vi "USRP Config.vi"(0 "USRP Configuration":T6={"USRP RIO Resources"=["USRP-2954"], "reference frequency source"="Internal"}, 5 "rx config":T4={"rf enable 0"=FALSE, "rf config 0"={"antenna"="RX2", "frequency"=2000000000.0, "lo frequency"=-1.0, "level"=0.0}, "rf enable 1"=FALSE, "rf config 1"={"antenna"="RX2", "frequency"=2000000000.0, "lo frequency"=-1.0, "level"=0.0}, "transfer mode"=enum."Finite", "sample rate"=10000000.0, "start trigger"=enum."Immediate"} {"sample rate" format="%#.3pS/s"; "rf config 1"."level" format="%#_gdBm"; "rf config 1"."lo frequency" format="%#.3pHz"; "rf config 1"."frequency" format="%#.3pHz"; "rf config 0"."level" format="%#_gdBm"; "rf config 0"."lo frequency" format="%#.3pHz"; "rf config 0"."frequency" format="%#.3pHz"}, 7 "tx config":T3={"rf enable 0"=FALSE, "rf config 0"={"antenna"="TX1", "frequency"=2000000000.0, "lo frequency"=-1.0, "level"=0.0}, "rf enable 1"=FALSE, "rf config 1"={"antenna"="TX1", "frequency"=2000000000.0, "lo frequency"=-1.0, "level"=0.0}, "transfer mode"=enum."Finite", "sample rate"=10000000.0, "start trigger"=enum."Immediate"} {"sample rate" format="%#.3pS/s"; "rf config 0"."level" format="%#_gdBm"; "rf config 0"."lo frequency" format="%#.3pHz"; "rf config 0"."frequency" format="%#.3pHz"; "rf config 1"."level" format="%#_gdBm"; "rf config 1"."lo frequency" format="%#.3pHz"; "rf config 1"."frequency" format="%#.3pHz"}, 11 "error in (no error)":errorcluster, 12 "Rx?":bool) -> (2 "tx channels":T1={"tx config"={"channel configuration"=[{"channel enable"=FALSE, "channel configuration"={"antenna"="TX1", "frequency"=2000000000.0, "lo frequency"=-1.0, "level"=0.0}}, {"channel enable"=FALSE, "channel configuration"={"antenna"="TX1", "frequency"=2000000000.0, "lo frequency"=-1.0, "level"=0.0}}], "transfer mode"=enum."Finite", "sample rate"=10000000.0, "number of samples"=8192, "start trigger"=enum."Immediate", "tone frequency"=100000.0}, "reference frequency source"="Internal", "tx.data source"=enum."SFP Port 1", "tx.enabled channels"=[], "I"=[], "Q"=[], "tx.coerced configurations"={"coerced frequencies"=[], "coerced lo frequencies"=[], "coerced levels"=[], "coerced sample rates"=[]}} {"tx.coerced configurations"."coerced sample rates" format="%#.3pS/s"; "tx.coerced configurations"."coerced levels" format="%#.3gdBm"; "tx.coerced configurations"."coerced lo frequencies" format="%#.3pHz"; "tx.coerced configurations"."coerced frequencies" format="%#.3pHz"; "tx config"."channel configuration"."channel configuration"."frequency" format="%#.3pHz"; "tx config"."channel configuration"."channel configuration"."lo frequency" format="%#.3pHz"; "tx config"."channel configuration"."channel configuration"."level" format="%#_gdBm"; "tx config"."tone frequency" format="%#.3pHz"; "tx config"."sample rate" format="%#.3pS/s"}, 3 "tx.enabled channels":string[][](array[string]), 4 "niUsrpRio Session":T8[](array[typedef]) {"Daughterboard Clock Rate" format="%#.3pHz"; "FPGA Data Clock Rate" format="%#.3pHz"; "Data Clock Rate" format="%#.3pHz"; "Characterization Data"."Frequencies [Hz]" format="%#_6p"; "EEPROM Characterization Header"."Pointer to Device Data Header" format="%x"; "EEPROM Characterization Header"."Checksum" format="%x"; "Device Data Header"."Pointer to Characterization Data" format="%x"; "Device Data Header"."Checksum" format="%x"; "EEPROM Header"."Pointer to User Header" format="%x"; "EEPROM Header"."Pointer to Factory Header" format="%x"; "EEPROM Header"."Product Code" format="%x"; "EEPROM Header"."Checksum" format="%x"}, 6 "start trigger out":T2=enum."Immediate", 8 "USRP RIO Ports":bool[](array[boolean]), 10 "Time Stamp":timestamp=timestamp(5 s since 1904-01-01), 13 "rx channels":T5={"rx config"={"channel configuration"=[{"channel enable"=TRUE, "channel configuration"={"antenna"="RX2", "frequency"=2000000000.0, "lo frequency"=-1.0, "level"=0.0}}, {"channel enable"=TRUE, "channel configuration"={"antenna"="RX2", "frequency"=2000000000.0, "lo frequency"=-1.0, "level"=0.0}}], "transfer mode"=enum."Finite", "sample rate"=10000000.0, "number of samples"=8192, "start trigger"=enum."Immediate"}, "reference frequency source"="Internal", "rx.data sink"=enum."SFP Port 0", "rx.enabled channels"=["rx/RF 0"], "vertical range"=[0.29773949633541547], "rx.coerced configurations"={"coerced frequencies"=[2000000000.0], "coerced lo frequencies"=[2000000000.0], "coerced levels"=[-6.54387092590332], "coerced sample rates"=[10000000.000000853]}} {"rx.coerced configurations"."coerced sample rates" format="%#.3pS/s"; "rx.coerced configurations"."coerced levels" format="%#.3gdBm"; "rx.coerced configurations"."coerced lo frequencies" format="%#.3pHz"; "rx.coerced configurations"."coerced frequencies" format="%#.3pHz"; "rx config"."channel configuration"."channel configuration"."frequency" format="%#.3pHz"; "rx config"."channel configuration"."channel configuration"."lo frequency" format="%#.3pHz"; "rx config"."channel configuration"."channel configuration"."level" format="%#_gdBm"; "rx config"."sample rate" format="%#.3pS/s"; "vertical range" format="%#.3pVpp"}, 14 "rx.enabled channels":string[][](array[string])=[["rx/RF 0"]], 15 "error out":errorcluster={"status"=TRUE, "code"=-61206, "source"="Configure Stream.vi"})   [LabVIEW 2016]
uses:
  <instrlib>/niUsrpRio/Config/v1/Host/Public/niUsrpRio Session.ctl
  <instrlib>/_niInstr/Register Bus/v0/Host/Public/Register Bus Session.ctl
  <instrlib>/_niInstr/Register Bus/v0/Host/Private/Session Data.ctl
  <instrlib>/niUsrpRio/Config/v1/Host/Private/DB Queue Reference.ctl
  <instrlib>/niUsrpRio/Config/v1/Host/Private/Daughterboard Data.ctl
  <instrlib>/niUsrpRio/Config/v1/Host/Private/ATR state data.ctl
  <instrlib>/niUsrpRio/Config/v1/Host/Private/Antenna Configuration.ctl
  <instrlib>/niUsrpRio/Config/v1/Host/Private/CPLD Power Mode.ctl
  <instrlib>/niUsrpRio/Config/v1/Host/Public/EEPROM Header.ctl
  <instrlib>/niUsrpRio/Config/v1/Host/Public/EEPROM Device Data Header.ctl
  <instrlib>/niUsrpRio/Config/v1/Host/Public/EEPROM Characterization Header.ctl
  <instrlib>/niUsrpRio/Config/v1/Host/Public/Characterization Data.ctl
  <instrlib>/niUsrpRio/Config/v1/Host/Public/IQ Imbalance.ctl
  2954/SubVIs/Start Trigger.ctl
  TypeDefs/USRP Configuration.ctl
  <vilib>/userdefined/Silver/nirio_resource_slv.ctl
  2954/SubVIs/Rx Channels.ctl
  TypeDefs/Rx Config.ctl
  TypeDefs/Tx Config.ctl
  2954/SubVIs/Tx Channels.ctl
  <instrlib>/_niInstr/Register Bus/v0/Host/niInstr Register Bus v0 Host.lvlib
  <instrlib>/niUsrpRio/Config/v1/Host/niUsrpRio Config v1 Host.lvlib
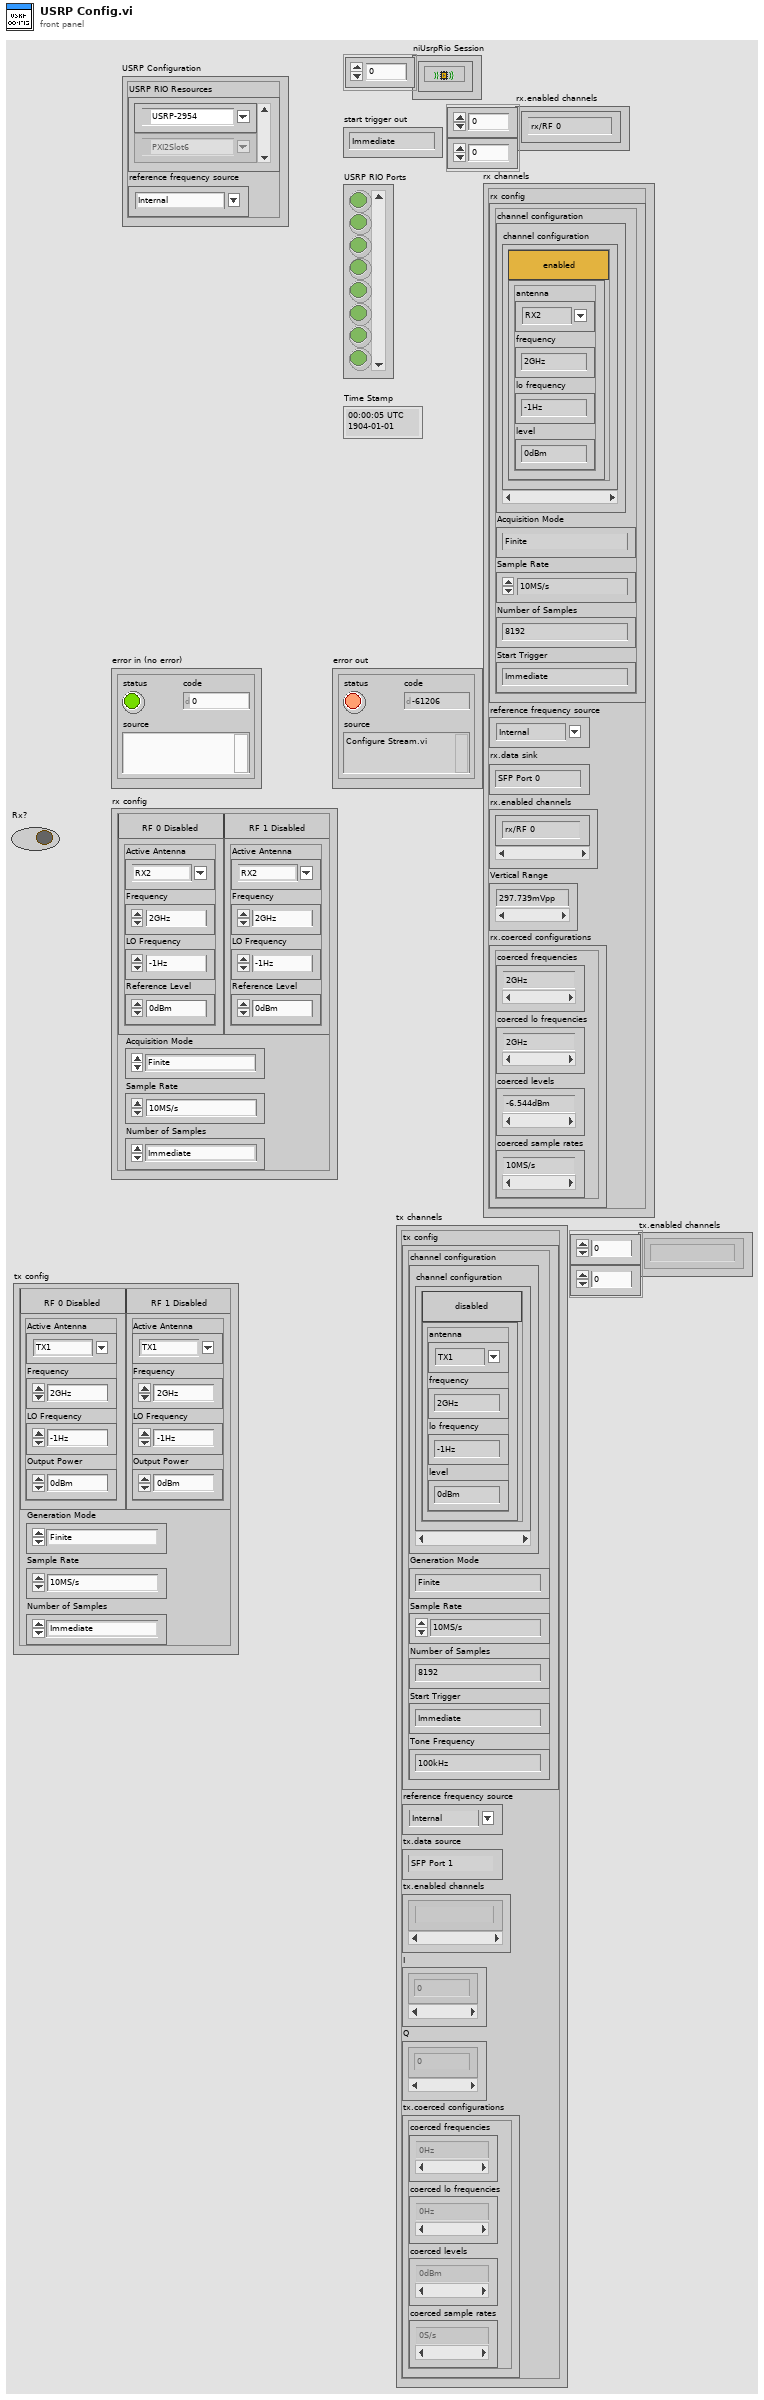
[diagram p1: front panel]
types:
  T1 = typedef "Tx Channels.ctl" = cluster{"tx config":cluster{"channel configuration":cluster{"channel enable":bool, "channel configuration":cluster{"antenna":string, "frequency":dbl, "lo frequency":dbl, "level":dbl}}[], "transfer mode":enum16{"Finite", "Continuous"}, "sample rate":dbl, "number of samples":u32, "start trigger":T2, "tone frequency":dbl}, "reference frequency source":string, "tx.data source":enum16{"SFP Port 0", "SFP Port 1", "Host"}, "tx.enabled channels":string[], "I":i16[], "Q":i16[], "tx.coerced configurations":cluster{"coerced frequencies":dbl[], "coerced lo frequencies":dbl[], "coerced levels":dbl[], "coerced sample rates":dbl[]}}
  T2 = typedef "Start Trigger.ctl" = enum8{"Software", "Digital Edge", "Rx Start Trigger", "Tx Start Trigger", "Immediate", "Future Time Event"}
  T3 = typedef "Tx Config.ctl" = cluster{"rf enable 0":bool, "rf config 0":cluster{"antenna":string, "frequency":dbl, "lo frequency":dbl, "level":dbl}, "rf enable 1":bool, "rf config 1":cluster{"antenna":string, "frequency":dbl, "lo frequency":dbl, "level":dbl}, "transfer mode":enum16{"Finite", "Continuous"}, "sample rate":dbl, "start trigger":T2}
  T4 = typedef "Rx Config.ctl" = cluster{"rf enable 0":bool, "rf config 0":cluster{"antenna":string, "frequency":dbl, "lo frequency":dbl, "level":dbl}, "rf enable 1":bool, "rf config 1":cluster{"antenna":string, "frequency":dbl, "lo frequency":dbl, "level":dbl}, "transfer mode":enum16{"Finite", "Continuous"}, "sample rate":dbl, "start trigger":T2}
  T5 = typedef "Rx Channels.ctl" = cluster{"rx config":cluster{"channel configuration":cluster{"channel enable":bool, "channel configuration":cluster{"antenna":string, "frequency":dbl, "lo frequency":dbl, "level":dbl}}[], "transfer mode":enum16{"Finite", "Continuous"}, "sample rate":dbl, "number of samples":u32, "start trigger":T2}, "reference frequency source":string, "rx.data sink":enum16{"SFP Port 0", "SFP Port 1", "Host"}, "rx.enabled channels":string[], "vertical range":dbl[], "rx.coerced configurations":cluster{"coerced frequencies":dbl[], "coerced lo frequencies":dbl[], "coerced levels":dbl[], "coerced sample rates":dbl[]}}
  T6 = typedef "USRP Configuration.ctl" = cluster{"USRP RIO Resources":T7[], "reference frequency source":string}
  T7 = typedef "nirio_resource_slv.ctl" = tag
  T8 = typedef "niUsrpRio Config v1 Host.lvlib/niUsrpRio Session.ctl" = cluster{"FPGA Interface":refnum<k20>, "RIO Interface Number":u32, "Data Clock Rate":u32, "FPGA Data Clock Rate":u32, "Global Settings Register Bus":T9, "Radio 0 Settings Register Bus":T9, "Radio 1 Settings Register Bus":T9, "Radio Settings Bus Semaphore":T10, "DB Queues":T11[], "Characterization Data Valid?":bool, "EEPROM Header":T12, "Device Data Header":T13, "EEPROM Characterization Header":T14, "Characterization Data":T15[], "FPGA Current Version":u32, "FPGA Oldest Compatible Version":u32, "Fixed Logic Current Version":u32, "Fixed Logic Oldest Compatible Version":u32, "FPGA Radio Settings Bus Current Version":u32, "FPGA Radio Settings Bus Oldest Compatible Version":u32, "FPGA Board Config Current Version":u32, "FPGA Board Config Oldest Compatible Version":u32, "Daughterboard Clock Rate":u32, "daughterboard configuration session handles":u64[]}
  T9 = typedef "niInstr Register Bus v0 Host.lvlib/Register Bus Session.ctl" = refnum<queue>
  T10 = typedef "Semaphore RefNum" = refnum<k1>
  T11 = typedef "niUsrpRio Config v1 Host.lvlib/DB Queue Reference.ctl" = refnum<queue>
  T12 = typedef "niUsrpRio Config v1 Host.lvlib/EEPROM Header.ctl" = cluster{"Checksum":u32, "Product Code":u16, "Hardware Current Version":u16, "Hardware Oldest Compatible Version":u16, "EEPROM Map Current Version":u16, "EEPROM Map Oldest Compatible Version":u16, "User Password":string, "Pointer to Factory Header":u32, "Pointer to User Header":u32, "Recommended Interval":u16, "Number of Reserved Bytes":i32, "Number of Daughterboards":u8, "Daughterboard IDs":u16[], "Daughterboard Serial Numbers":string[]}
  T13 = typedef "niUsrpRio Config v1 Host.lvlib/EEPROM Device Data Header.ctl" = cluster{"Checksum":u32, "Number of Channels":u8, "Number of Gain Settings":u16[], "Pointer to Characterization Data":u32[], "Number of Reserved Bytes":i32, "Number of Frequencies":u16[]}
  T14 = typedef "niUsrpRio Config v1 Host.lvlib/EEPROM Characterization Header.ctl" = cluster{"Checksum":u32, "Date":timestamp, "Temperature":sgl, "Misc. Info":string, "Pointer to Device Data Header":u32, "Number of Reserved Bytes":i32}
  T15 = typedef "niUsrpRio Config v1 Host.lvlib/Characterization Data.ctl" = cluster{"Gains[dB]":dbl[], "Frequencies [Hz]":dbl[], "IQ Imbalance Table":T16[], "Measured Gains[dB]":dbl[][]}
  T16 = typedef "niUsrpRio Config v1 Host.lvlib/IQ Imbalance.ctl" = cluster{"Gain Imbalance [linear]":dbl, "Phase Imbalance [radians]":dbl, "Offset":cdb}
  T17 = cluster{"channel configuration":cluster{"channel enable":bool, "channel configuration":cluster{"antenna":string, "frequency":dbl, "lo frequency":dbl, "level":dbl}}[], "transfer mode":enum16{"Finite", "Continuous"}, "sample rate":dbl, "number of samples":u32, "start trigger":T2, "tone frequency":dbl}
  T18 = cluster{"channel configuration":cluster{"channel enable":bool, "channel configuration":cluster{"antenna":string, "frequency":dbl, "lo frequency":dbl, "level":dbl}}[], "transfer mode":enum16{"Finite", "Continuous"}, "sample rate":dbl, "number of samples":u32, "start trigger":T2}
  T19 = cluster{"hard error":bool, "soft error":bool, "lane up":bool, "channel up":bool, "sys reset":bool}[]
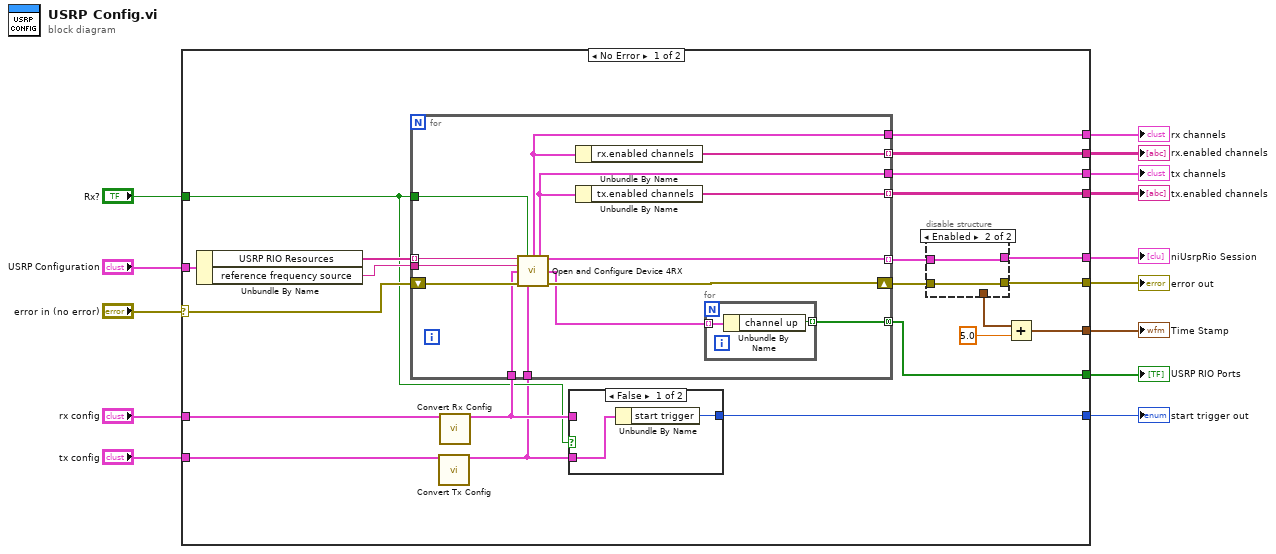
[diagram p0: block diagram]
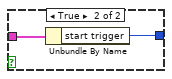
[diagram p2: hidden frame]
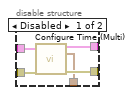
[diagram p3: hidden frame]
diagram:
  n1 = case shown="No Error" "error in (no error)" {
    selector: "error in (no error)" -> [w21 w64]
    tunnel: [w34 _] -> w14
    tunnel: [w33 w64] -> w13
    tunnel: [w31 _] -> w12
    tunnel: [w30 _] -> w11
    tunnel: [w26 _] -> w10
    tunnel: [w25 _] -> w9
    tunnel: [w24 _] -> w8
    tunnel: "USRP Configuration" -> [w22 _]
    tunnel: "rx config" -> [w15 _]
    tunnel: "tx config" -> [w18 _]
    tunnel: [w20 _] -> w3
    tunnel: [w19 _] -> w2
    tunnel: "Rx?" -> [w17 _]
    frame No Error {
      n2 = Unbundle By Name(w22) -> ("USRP RIO Resources"=w28:T7[], "reference frequency source"=w27:string)
      n3 = call "Convert Tx Config.vi"("tx config"=w18) -> ("tx config out"=w16:T17)  [unwired: 14 in]
      n4 = call "Convert Rx Config.vi"("rx config"=w15) -> ("rx config out"=w23:T18)  [unwired: 14 in]
      n5 = for {
        tunnel: w27 -> [w55]
        tunnel: w28 -> [w61] mode=indexing
        shift-right: [w59] -> w32
        shift-left: w21 -> [w60]
        tunnel: [w58] -> w36 mode=indexing
        tunnel: [w56] -> w31 mode=concatenating
        tunnel: [w54] -> w26 mode=indexing
        tunnel: [w53] -> w25
        tunnel: w23 -> [w52]
        tunnel: w16 -> [w51]
        tunnel: [w50] -> w20
        tunnel: [w49] -> w19 mode=indexing
        tunnel: w17 -> [w48]
        n6 = call "Open and Configure Device 4RX.vi"("USRP RIO Device"=w61, "Rx?"=w48, "reference frequency source"=w55, "rx config"=w52, "error in"=w60, "tx config"=w51) -> ("rx channels"=w53:T5, "tx channels"=w50:T1, "niUsrpRio Session (out)"=w58:T8, "Ports debug"=w57:T19, "error out"=w59:errorcluster)  [unwired: 4 in, 1 out]
        n7 = Unbundle By Name(w53) -> ("rx.enabled channels"=w54:string[])
        n8 = Unbundle By Name(w50) -> ("tx.enabled channels"=w49:string[])
        n9 = for {
          tunnel: w57 -> [w63] mode=indexing
          tunnel: [w62] -> w56 mode=indexing
          n10 = Unbundle By Name(w63) -> ("channel up"=w62:bool)
        }
      }
      n11 = case shown="False" w17 {
        tunnel: [w37 w40] -> w24
        tunnel: w23 -> [_ w39]
        tunnel: w16 -> [w38 _]
        frame False {
          n12 = Unbundle By Name(w38) -> ("start trigger"=w37:T2)
        }
        frame True {
          n13 = Unbundle By Name(w39) -> ("start trigger"=w40:T2)
        }
      }
      n14 = disable-structure shown="Enabled" {
        disable-tunnel: w36 -> [w45 w47]
        disable-tunnel: w32 -> [w44 w46]
        disable-tunnel: [w43 w46] -> w33
        disable-tunnel: [w42 w47] -> w34
        disable-tunnel: [w41 _] -> w35
        frame Disabled {
          n15 = call "Configure Time (Multi).vi"("niUsrpRio Sessions"=w45, "error in"=w44) -> ("niUsrpRio Sessions (out)"=w42:T8[], "time"=w41:timestamp, "error out"=w43:errorcluster)  [unwired: 11 in]
        }
        frame Enabled {
        }
      }
      n16 = Add(x=w35, y=5.0) -> (x+y=w30:timestamp)
    }
    frame Error {
    }
  }
  "USRP RIO Ports" <- w12
  "niUsrpRio Session" <- w14
  "error out" <- w13
  "Time Stamp" <- w11
  "start trigger out" <- w8
  "rx.enabled channels" <- w10
  "rx channels" <- w9
  "tx channels" <- w3
  "tx.enabled channels" <- w2
